vi "Increment Name.vi"(1 "Sample Name":string) -> (0 "Sample Name 2":string)   [LabVIEW 2012]
doc: "Increment or add a number to a string name. \nIE Temperature Test -> Temperature Test 2\nSample A22 -> Sample A23"
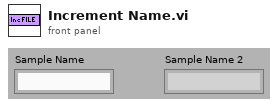
[diagram p1: front panel]
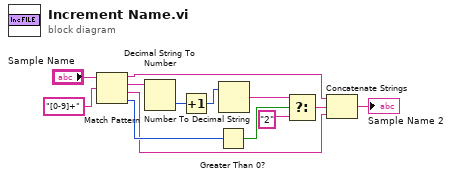
[diagram p0: block diagram]
diagram:
  n1 = Match Pattern(string="Sample Name", regular expression="[0-9]+") -> (before substring=w6:string, match substring=w5:string, after substring=w1:string, offset past match=w3:i32)  [unwired: 1 in]
  n2 = Decimal String To Number(string=w5) -> (number=w10:i32)  [unwired: 2 in, 1 out]
  n3 = Increment(x=w10) -> (x+1=w11:i32)
  n4 = Greater Than 0?(x=w3) -> (x > 0?=w9:bool)
  n5 = Number To Decimal String(number=w11) -> (decimal integer string=w12:string)  [unwired: 1 in]
  n6 = Select(t=w12, s=w9, f="2" ("string")) -> (s? t:f=w8:string)
  n7 = Concatenate Strings(w6, w8, w1) -> (→"Sample Name 2":string)
